vi "CreateSPICommand.vi"(7 "Write/Read":bool, 10 "Write Value":u8[](array[numeric]) format="%.0x", 11 "Register Address":u8[](array[numeric]) format="%.0x") -> (2 "Command Value":u32[](array[numeric]), 3 "Command Bitstream":bool[][](array[boolean]))   [LabVIEW 2023]
panel:
  # "!"
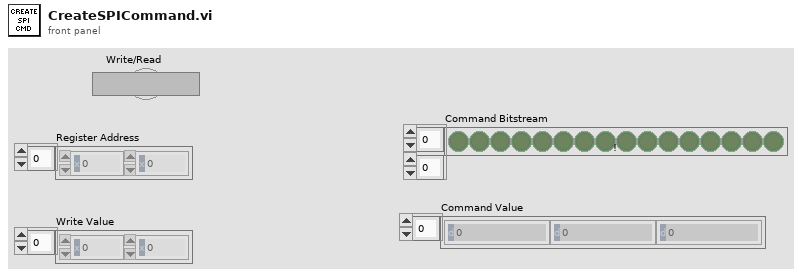
[diagram p1: front panel]
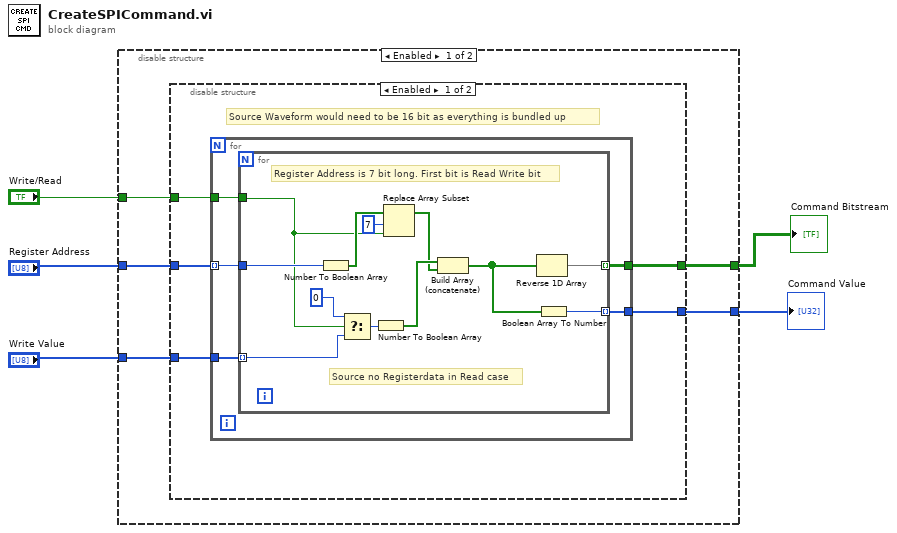
[diagram p0: block diagram]
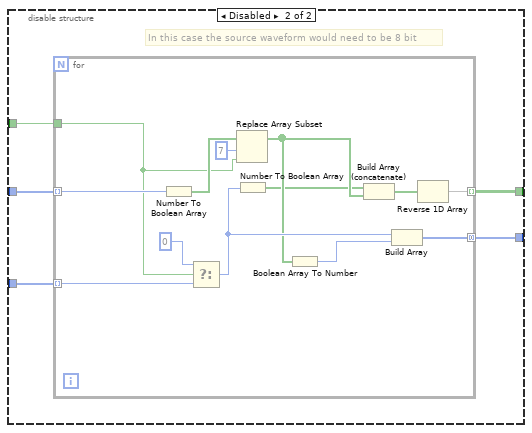
[diagram p2: hidden frame]
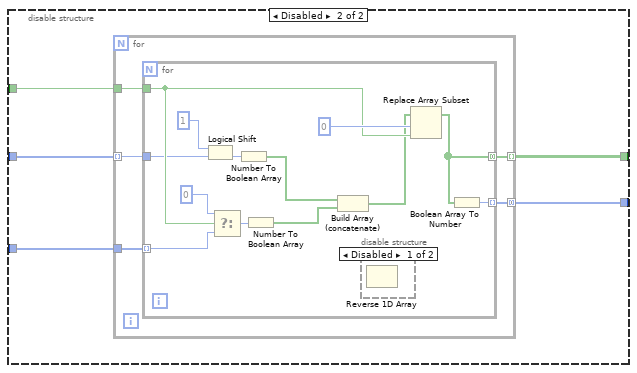
[diagram p3: hidden frame]
diagram:
  n1 = disable-structure shown="Enabled" {
    disable-tunnel: [w10 w51] -> w5
    disable-tunnel: "Write Value" -> [w9 w54]
    disable-tunnel: "Register Address" -> [w8 w55]
    disable-tunnel: "Write/Read" -> [w7 w53]
    disable-tunnel: [w6 w52] -> w2
    frame Enabled {
      n2 = disable-structure shown="Enabled" {
        disable-tunnel: [w15 w33] -> w10
        disable-tunnel: w9 -> [w14 w37]
        disable-tunnel: w8 -> [w13 w35]
        disable-tunnel: w7 -> [w12 w36]
        disable-tunnel: [w11 w34] -> w6
        frame Enabled {
          # "Source Waveform would need to be 16 bit as everything is bundled up"
          n3 = for {
            tunnel: [w20] -> w15
            tunnel: w14 -> [w19]
            tunnel: w13 -> [w18] mode=indexing
            tunnel: w12 -> [w17]
            tunnel: [w16] -> w11
            n4 = for {
              tunnel: w18 -> [w32]
              tunnel: w19 -> [w28] mode=indexing
              tunnel: [w30] -> w20 mode=indexing
              tunnel: [w29] -> w16 mode=indexing
              tunnel: w17 -> [w24]
              # "Register Address is 7 bit long. First bit is Read Write bit"
              # "Source no Registerdata in Read case"
              n5 = Number To Boolean Array(number=w32) -> (Boolean array=w25:bool[])
              n6 = Select(t=u8 0, s=w24, f=w28) -> (s? t:f=w27:u8)
              n7 = Number To Boolean Array(number=w27) -> (Boolean array=w31:bool[])
              n8 = Replace Array Subset(array=w25, new element=w24, index=7) -> (w22:bool[])
              n9 = Build Array (concatenate)(w31, w22) -> (w21:bool[])
              n10 = Reverse 1D Array(array=w21) -> (reversed array=w30:bool[])
              n11 = Boolean Array To Number(Boolean array=w21) -> (number=w29:u32)
            }
          }
        }
        frame Disabled {
          # "In this case the source waveform would need to be 8 bit"
          n12 = for {
            tunnel: w37 -> [w49] mode=indexing
            tunnel: w36 -> [w45]
            tunnel: w35 -> [w46] mode=indexing
            tunnel: [w42] -> w34 mode=concatenating
            tunnel: [w38] -> w33 mode=indexing
            n13 = Number To Boolean Array(number=w46) -> (Boolean array=w48:bool[])
            n14 = Select(t=u8 0, s=w45, f=w49) -> (s? t:f=w44:u8)
            n15 = Replace Array Subset(array=w48, new element=w45, index=7) -> (w41:bool[])
            n16 = Number To Boolean Array(number=w44) -> (Boolean array=w40:bool[])
            n17 = Boolean Array To Number(Boolean array=w41) -> (number=w43:u32)
            n18 = Build Array (concatenate)(w40, w41) -> (w39:bool[])
            n19 = Build Array(w44, w43) -> (w42:u32[])
            n20 = Reverse 1D Array(array=w39) -> (reversed array=w38:bool[])
          }
        }
      }
    }
    frame Disabled {
      n21 = for {
        tunnel: w55 -> [w58] mode=indexing
        tunnel: w54 -> [w60]
        tunnel: w53 -> [w59]
        tunnel: [w57] -> w52 mode=concatenating
        tunnel: [w56] -> w51 mode=indexing
        n22 = for {
          tunnel: w60 -> [w69] mode=indexing
          tunnel: w59 -> [w70]
          tunnel: w58 -> [w63]
          tunnel: [w66] -> w57 mode=indexing
          tunnel: [w65] -> w56 mode=concatenating
          n23 = Logical Shift(y=i16 1, x=w63) -> (x << y=w61:u8)
          n24 = Select(t=u8 0, s=w70, f=w69) -> (s? t:f=w72:u8)
          n25 = Number To Boolean Array(number=w61) -> (Boolean array=w67:bool[])
          n26 = Number To Boolean Array(number=w72) -> (Boolean array=w68:bool[])
          n27 = Build Array (concatenate)(w67, w68) -> (w64:bool[])
          n28 = disable-structure shown="Disabled" {
            frame Disabled {
              n29 = Reverse 1D Array() -> ()  [unwired: 1 in, 1 out]
            }
            frame Enabled {
            }
          }
          n30 = Replace Array Subset(array=w64, new element=w70, index=0) -> (w65:bool[])
          n31 = Boolean Array To Number(Boolean array=w65) -> (number=w66:u32)
        }
      }
    }
  }
  "Command Bitstream" <- w5
  "Command Value" <- w2
